vi "Acquire Pulse Result.vi"(8 "error in (no error)":errorcluster, 11 "Pulse Recorder Actor in":refnum<class "Pulse Recorder Actor.lvclass">) -> (0 "error out":errorcluster, 2 "Pulse acquired":bool, 3 "Pulse Recorder Actor out":refnum<class "Pulse Recorder Actor.lvclass">)   [LabVIEW 2021, in "Pulse Recorder Actor.lvclass"]
uses:
  Pulse Recorder Actor.lvclass
  C:/GitHub/LabActor/Template Module/Template Module.lvclass
  C:/Program Files/National Instruments/LabVIEW 2021/vi.lib/ActorFramework/Actor/Actor.lvclass
  Template Module/Template Module.lvclass/Template Module.ctl
  Publish-Subscribe/Context.ctl
  NHMFL_Core/Libraries/Instruments/Results/Acquired Result/Acquired Result.lvclass
  C:/GitHub/LabActor/Publish-Subscribe/Interfaces/Information/Information.lvclass
  Controllers/Process Controller/Request type.ctl
  <vilib>/ActorFramework/Actor/Actor.lvclass/Actor.ctl
  Publish-Subscribe/Interfaces/Subscriber Messages/Information Msg/Information Msg.lvclass/Information Msg.ctl
  <vilib>/ActorFramework/Message Enqueuer/Message Enqueuer.lvclass/Message Enqueuer.ctl
  Template Module/Read Name.vi
  <vilib>/ActorFramework/Message Enqueuer/Enqueue.vi
  Publish-Subscribe/Interfaces/Subscriber Messages/Information Msg/Information Msg.lvclass
  C:/Program Files/National Instruments/LabVIEW 2021/vi.lib/ActorFramework/Message/Message.lvclass
  Read Pulse driver.vi
  Write Pulse driver.vi
  <vilib>/ActorFramework/Message Priority Queue/Priority Enqueue.vi
  NHMFL_Core/Libraries/Instruments/Pulse Driver/Pulse Driver.lvclass
  <vilib>/ActorFramework/Actor/Actor.lvclass
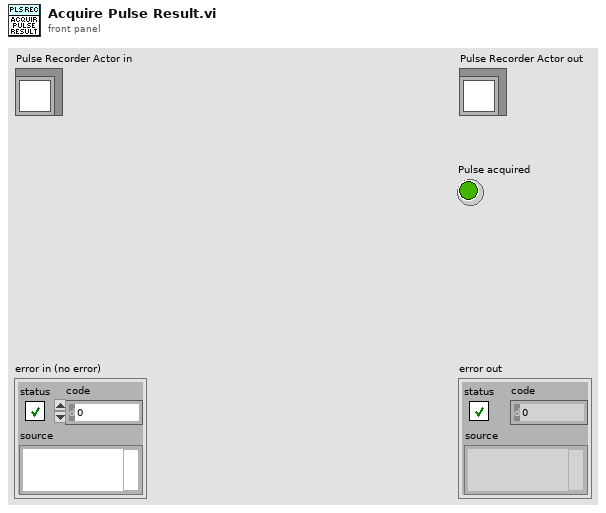
[diagram p1: front panel]
types:
  T1 = typedef "Request type.ctl" = enum16{"Process complete", "User command", "Auto-restart", "Error"}
  T2 = typedef "Context.ctl" = cluster{"Topic":string, "Source":string}
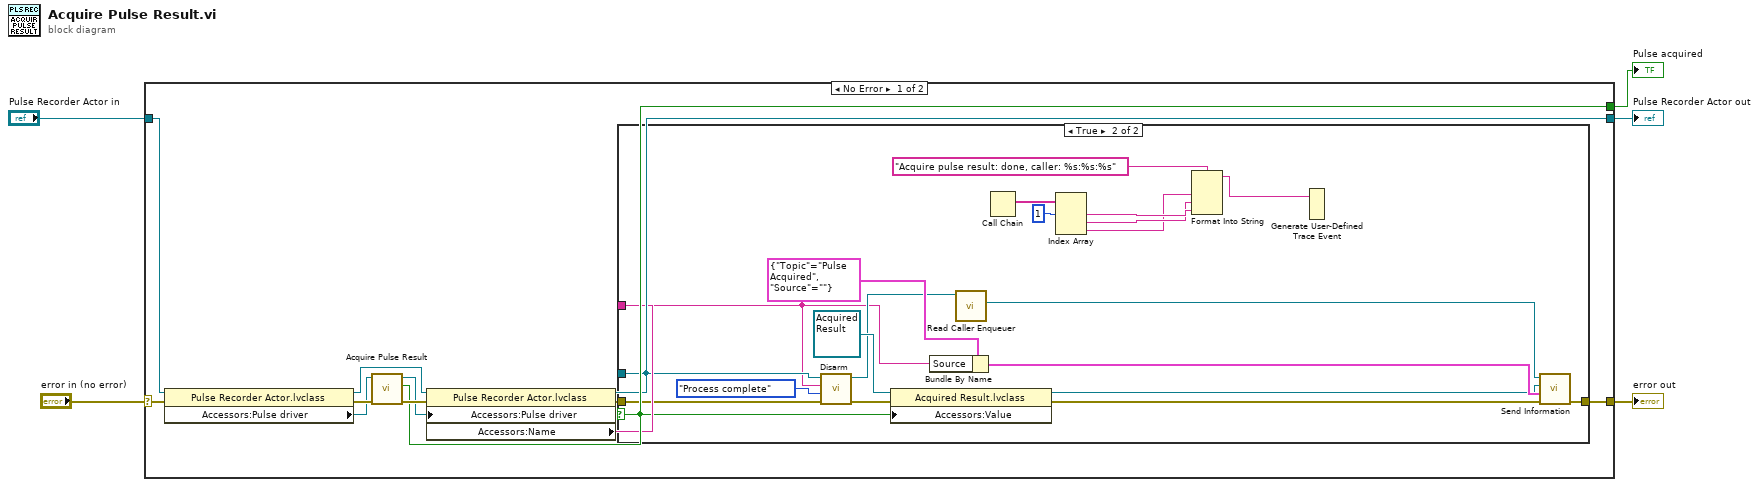
[diagram p0: block diagram]
diagram:
  n1 = case shown="No Error" "error in (no error)" {
    selector: "error in (no error)" -> [w17 w41]
    tunnel: [w6 w41] -> w4
    tunnel: [w8 w40] -> w2
    tunnel: "Pulse Recorder Actor in" -> [w16 w40]
    tunnel: [w9 _] -> w1
    frame No Error {
      n2 = property class="Pulse Recorder Actor.lvclass"(reference=w16, error in=w17) -> (reference out=w12:refnum<class "Pulse Recorder Actor.lvclass">, error out=w15:errorcluster, "Accessors:Pulse driver"=w11:refnum<class "Pulse Driver.lvclass">)
      n3 = call-dynamic "Acquire Pulse Result.vi"("error in (no error)"=w15, "Pulse Driver in"=w11) -> ("error out"=w14:errorcluster, "Pulse acquired"=w9:bool, "Pulse Driver out"=w13:refnum<class "Pulse Driver.lvclass">)  [unwired: 7 in]
      n4 = property class="Pulse Recorder Actor.lvclass"(reference=w12, error in=w14, "Accessors:Pulse driver"=w13) -> (reference out=w8:refnum<class "Pulse Recorder Actor.lvclass">, error out=w10:errorcluster, "Accessors:Name"=w7:string)
      n5 = case shown="True" w9 {
        selector: w9 -> [_ w32]
        tunnel: w8 -> [_ w28]
        tunnel: w10 -> [w18 w30]
        tunnel: [w18 w36] -> w6
        tunnel: w7 -> [_ w26]
        frame False {
        }
        frame True {
          n6 = call-dynamic "Disarm.vi"("error in (no error)"=w30, "Request type"=Request_type."Process complete", "Requester"=w26, "Pulse Recorder Actor in"=w28) -> ("error out"=w31:errorcluster, "Pulse Recorder Actor out"=w29:refnum<class "Pulse Recorder Actor.lvclass">)  [unwired: 6 in]
          n7 = property class="Acquired Result.lvclass"(reference=refnum<class "Acquired Result.lvclass"> refnum ("Acquired Result.lvclass"), error in=w31, "Accessors:Value"=w32) -> (reference out=w33:refnum<class "Acquired Result.lvclass">, error out=w34:errorcluster)
          n8 = Bundle By Name(cluster=T2 {"Topic"="Pulse Acquired", "Source"=""} ("Context"), "Source"=w26) -> (w39:T2)
          n9 = call <vilib>:"Read Caller Enqueuer.vi"("Actor"=w29) -> ("Caller Enqueuer"=w38:refnum<class "Message Enqueuer.lvclass">)  [unwired: 10 in]
          n10 = Call Chain() -> (call chain=w24:string[])
          n11 = Index Array(array=w24, index #1=1 ("index")) -> (element #1=w23:string, element #2=w22:string, element #3=w21:string)  [unwired: 2 in]
          n12 = Format Into String(format string="Acquire pulse result: done, caller: %s:%s:%s" ("string"), w21, w22, w23) -> (resulting string=w19:string)  [unwired: 2 in, 1 out]
          n13 = Generate User-Defined Trace Event(2:w19) -> ()  [unwired: 1 in]
          n14 = call "Send Information.vi"("error in (no error)"=w34, "Context"=w39, "Information"=w33, "Message Enqueuer"=w38) -> ("error out"=w36:errorcluster)  [unwired: 6 in, 1 out]
        }
      }
    }
    frame Error {
    }
  }
  "error out" <- w4
  "Pulse Recorder Actor out" <- w2
  "Pulse acquired" <- w1
